vi "Test PieChart.vi"() -> ()   [LabVIEW 2020, in "PieChart.lvclass"]
uses:
  PieChart.lvclass
  Pie Slice.ctl
panel:
  in  "Show/Hide Title":bool
  in  "Show/Hide Legend":bool
  in  "Selection":i32 min=-1 max=9
  out "Pie Chart":picture
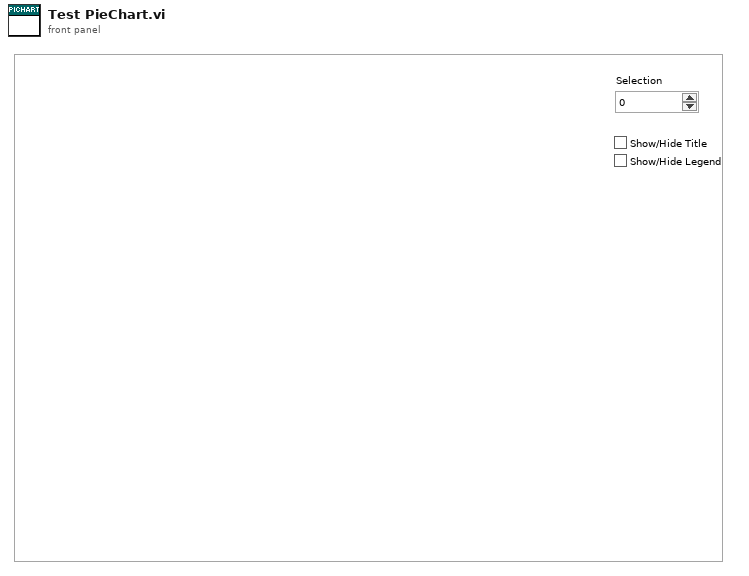
[diagram p1: front panel]
types:
  T1 = typedef "PieChart.lvclass/Pie Slice.ctl" = cluster{"Value":dbl, "Label":string}
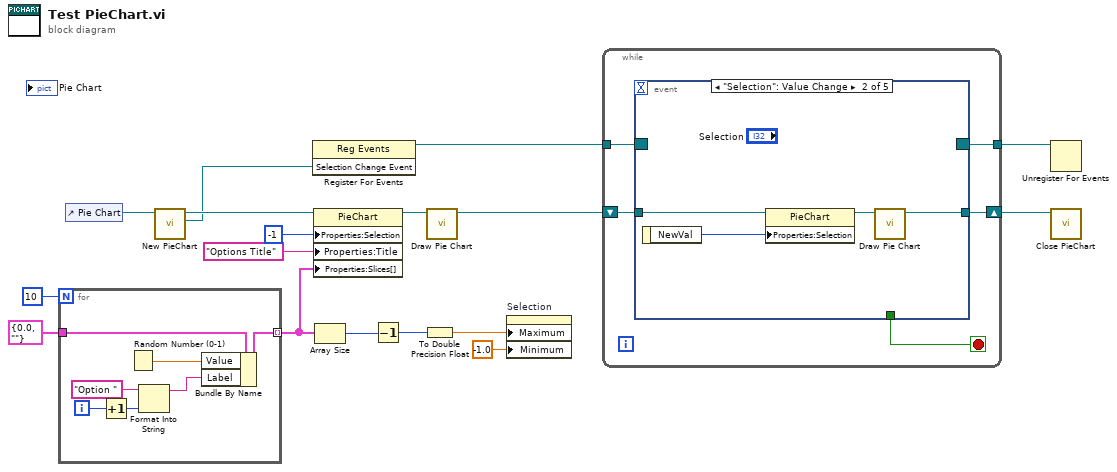
[diagram p0: block diagram]
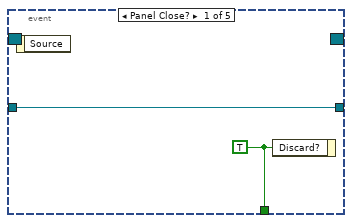
[diagram p2: hidden frame]
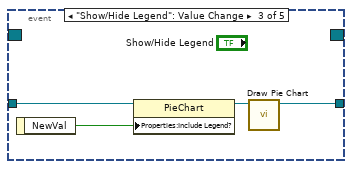
[diagram p3: hidden frame]
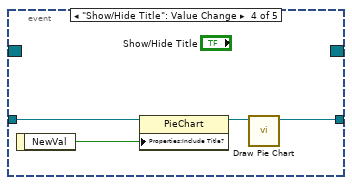
[diagram p4: hidden frame]
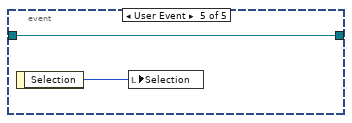
[diagram p5: hidden frame]
diagram:
  n1 = for {
    N: 10 -> [_]
    tunnel: T1 {"Value"=0.0, "Label"=""} ("Slice") -> [w24]
    tunnel: [w20] -> w5 mode=indexing
    i -> [w23]
    n2 = Increment(x=w23) -> (x+1=w22:i32)
    n3 = Random Number (0-1)() -> (number: 0 to 1=w19:dbl)
    n4 = Format Into String(initial string="Option ", w22) -> (resulting string=w18:string)  [unwired: 2 in, 1 out]
    n5 = Bundle By Name(cluster=w24, "Value"=w19, "Label"=w18) -> (w20:T1)
  }
  n6 = control-ref of="Pie Chart"() -> (w17:refnum<vi>)
  n7 = call "New PieChart.vi"("Reference"=w17) -> ("Selection Change Event"=w9:refnum<user-event>, "PieChart out"=w16:refnum<class "PieChart.lvclass">)  [unwired: 8 in, 1 out]
  n8 = register-events(w9) -> (reference out=w8:refnum<event-registration>)  [unwired: 2 in, 1 out]
  n9 = property class="PieChart"(reference=w16, "Properties:Selection"=-1 ("Selection"), "Properties:Title"="Options Title" ("Title"), "Properties:Slices[]"=w5) -> (reference out=w12:refnum<class "PieChart.lvclass">)  [unwired: 1 in, 1 out]
  n10 = Array Size(array=w5) -> (size(s)=w3:i32)
  n11 = Decrement(x=w3) -> (x-1=w1:i32)
  n12 = To Double Precision Float(number=w1) -> (double precision float=w2:dbl)
  n13 = call-dynamic "Draw Pie Chart.vi"("PieChart in"=w12) -> ("PieChart out"=w11:refnum<class "PieChart.lvclass">)  [unwired: 9 in, 1 out]
  n14 = property on="Selection" class="DigNum (strict)"("Maximum"=w2, "Minimum"=-1.0 ("Data Entry Limits:Minimum")) -> ()  [unwired: 2 in, 2 out]
  n15 = while {
    shift-right: [w28] -> w15
    shift-left: w11 -> [w27]
    tunnel: w8 -> [w26]
    tunnel: [w25] -> w7
    stop <- w29 stop-if-true
    n16 = event shown="[1] \"Selection\": Value Change" {
      selector: w26 -> [_ _ _ _ _]
      dyn-events: [_ _ _ _ _] -> w25
      timeout: _ -> [_ _ _ _ _]
      tunnel: [w31 _ _ _ _] -> w29
      tunnel: [w30 w33 w37 w41 w45] -> w28
      tunnel: w27 -> [w30 w35 w39 w43 w45]
      event Panel Close? {
        w31 = TRUE ("Discard?")
        n17 = event-data() -> ()  [unwired: 1 in, 1 out]
        n18 = event-data("Discard?"=w31) -> ()  [unwired: 1 in, 1 out]
      }
      event "Selection": Value Change {
        n19 = event-data() -> ("NewVal"=w32:i32)  [unwired: 1 in]
        n20 = property class="PieChart"(reference=w35, "Properties:Selection"=w32) -> (reference out=w34:refnum<class "PieChart.lvclass">)  [unwired: 1 in, 1 out]
        n21 = call-dynamic "Draw Pie Chart.vi"("PieChart in"=w34) -> ("PieChart out"=w33:refnum<class "PieChart.lvclass">)  [unwired: 9 in, 1 out]
      }
      event "Show/Hide Legend": Value Change {
        n22 = event-data() -> ("NewVal"=w36:bool)  [unwired: 1 in]
        n23 = property class="PieChart"(reference=w39, "Properties:Include Legend?"=w36) -> (reference out=w38:refnum<class "PieChart.lvclass">)  [unwired: 1 in, 1 out]
        n24 = call-dynamic "Draw Pie Chart.vi"("PieChart in"=w38) -> ("PieChart out"=w37:refnum<class "PieChart.lvclass">)  [unwired: 9 in, 1 out]
      }
      event "Show/Hide Title": Value Change {
        n25 = event-data() -> ("NewVal"=w40:bool)  [unwired: 1 in]
        n26 = property class="PieChart"(reference=w43, "Properties:Include Title?"=w40) -> (reference out=w42:refnum<class "PieChart.lvclass">)  [unwired: 1 in, 1 out]
        n27 = call-dynamic "Draw Pie Chart.vi"("PieChart in"=w42) -> ("PieChart out"=w41:refnum<class "PieChart.lvclass">)  [unwired: 9 in, 1 out]
      }
      event User Event {
        n28 = event-data() -> ("Selection"=w44:i32)  [unwired: 1 in]
        n29 = local write "Selection"(w44) -> ()
      }
    }
  }
  n30 = Unregister For Events(event registration refnum=w7) -> ()  [unwired: 1 in, 1 out]
  n31 = call "Close PieChart.vi"("PieChart in"=w15) -> ()  [unwired: 10 in, 1 out]
